vi "Set Transfers.vi"(10 "Transfers":refnum<class "Transfer.lvclass">[](array[class]), 11 "Transfer Group in":refnum<class "Transfer Group.lvclass">) -> (3 "Transfer Group out":refnum<class "Transfer Group.lvclass">)   [LabVIEW 2017, in "DSF Core.lvlib" / "Transfer Group.lvclass"]
uses:
  Transfer Group.lvclass
  Transfer/Transfer.lvclass
  Transfer Group.lvclass/Transfer Group.ctl
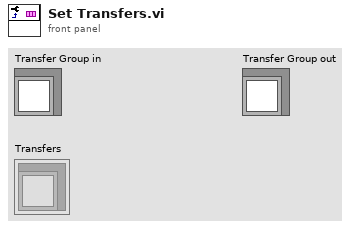
[diagram p1: front panel]
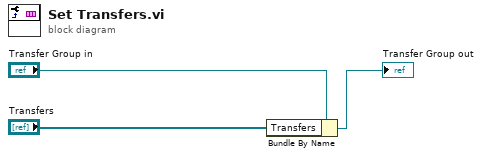
[diagram p0: block diagram]
diagram:
  n1 = Bundle By Name(cluster="Transfer Group in", "Transfers"="Transfers") -> (→"Transfer Group out":refnum<class "Transfer Group.lvclass">)
